vi "Create WaitForNotifier.vi"(10 "Wait until finished?":bool) -> (2 "Wait until finished? (dup)":bool, 3 "notifier":refnum<notifier>)   [LabVIEW 2021, in "BluePlot.lvlib"]
uses:
  BluePlot.lvlib
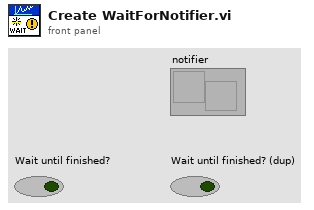
[diagram p1: front panel]
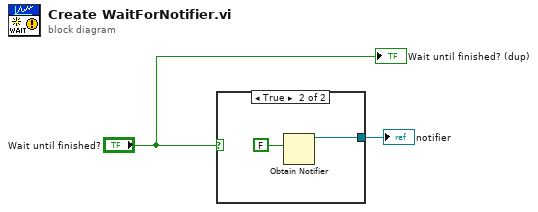
[diagram p0: block diagram]
diagram:
  n1 = case shown="True" "Wait until finished?" {
    tunnel: [_ w3] -> w2
    frame False {
    }
    frame True {
      n2 = Obtain Notifier(notification data type=FALSE) -> (notifier out=w3:refnum<notifier>)  [unwired: 3 in, 2 out]
    }
  }
  "notifier" <- w2
  "Wait until finished? (dup)" <- "Wait until finished?"
